vi "VdPhilipsMM-123_Create.vi"(8 "error in (no error)":errorcluster, 11 "reference in":refnum<class "VdPhilipsMM-123.lvclass">) -> (0 "error out":errorcluster, 3 "reference out":refnum<class "VdPhilipsMM-123.lvclass">)   [LabVIEW 2020, in "MulitMeters.lvlib" / "VdPhilipsMM-123.lvclass"]
uses:
  VdPhilipsMM-123.lvclass
  C:/Projects/DesignPatterns/StrategyPattern/VdMultiMeter_class/VdMultiMeter.lvclass
  VdPhilipsMM-123.lvclass/VdPhilipsMM-123.ctl
  VdMultiMeter_class/VdMultiMeter.lvclass
  C:/Projects/DesignPatterns/StrategyPattern/VdPhilipsMM-123_class/VdPhilipsMM-123.lvclass
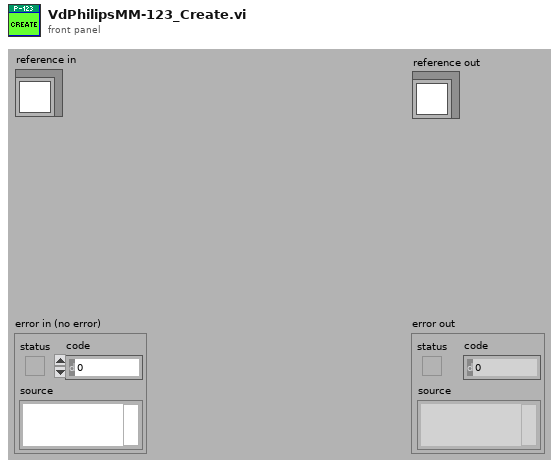
[diagram p1: front panel]
types:
  T1 = typedef "G4SubTemplate_Simple_4x4x4.lvclass/ObjectAttributes.ctl" = cluster{"Attribute1":dbl}
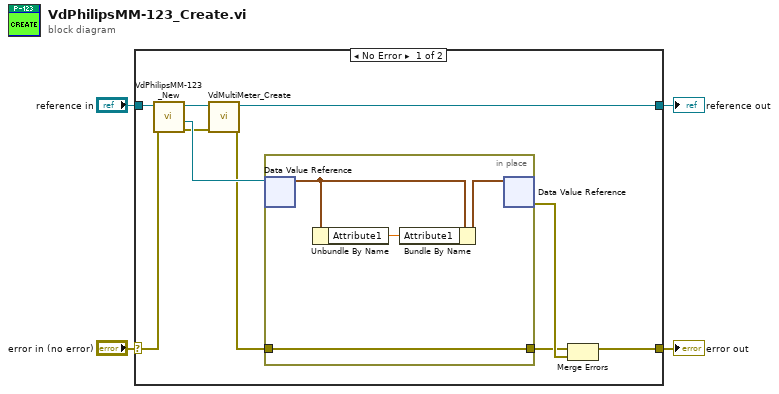
[diagram p0: block diagram]
diagram:
  n1 = case shown="No Error" "error in (no error)" {
    selector: "error in (no error)" -> [w10 w20]
    tunnel: [w8 w20] -> w3
    tunnel: "reference in" -> [w12 w19]
    tunnel: [w7 w19] -> w1
    frame No Error {
      n2 = call "VdPhilipsMM-123_New.vi"("error in (no error)"=w10, "reference in"=w12) -> ("error out"=w11:errorcluster, "DVRRefOut"=w14:refnum<data-value>, "reference out"=w13:refnum<class "VdPhilipsMM-123.lvclass">)  [unwired: 6 in, 1 out]
      n3 = call "VdMultiMeter_Create.vi"("error in (no error)"=w11, "reference in"=w13) -> ("error out"=w6:errorcluster, "reference out"=w7:refnum<class "VdPhilipsMM-123.lvclass">)  [unwired: 8 in]
      n4 = in-place {
        in-place-border: w6 -> [w15]
        in-place-border: [w15] -> w5
        n5 = in-place-dvr #1(w14) -> (w17:T1)  [unwired: 1 out]
        n6 = Unbundle By Name(w17) -> ("Attribute1"=w16:dbl)
        n7 = Bundle By Name(cluster=w17, "Attribute1"=w16) -> (w18:T1)
        n8 = in-place-dvr #1(w18) -> (w9:errorcluster)  [unwired: 1 out]
      }
      n9 = Merge Errors(w5, w9) -> (w8:errorcluster)
    }
    frame Error {
    }
  }
  "error out" <- w3
  "reference out" <- w1
